vi "Group Tags.vi"(8 "error in (no error)":errorcluster, 10 "Tag Names":string[](array[string]), 11 "Group":string) -> (0 "error out":errorcluster)   [LabVIEW 2010, in "Current Value Table.lvlib"]
doc: "This VI forms a named group which can be used to later read or write data to that entire group. This has the same functionality as including a set of groups during initialization. Tags can be members of multiple groups without issue."
uses:
  Current Value Table.lvlib
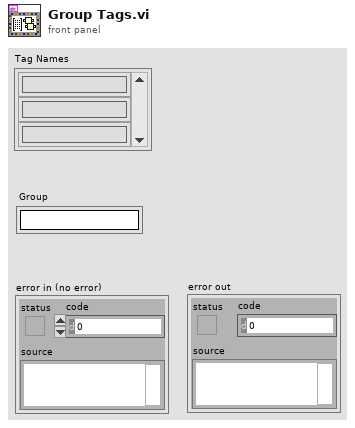
[diagram p1: front panel]
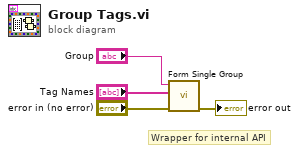
[diagram p0: block diagram]
diagram:
  # "Wrapper for internal API"
  n1 = call "Form Single Group.vi"("error in (no error)"="error in (no error)", "Names"="Tag Names", "Group"="Group") -> ("error out"=→"error out":errorcluster)  [unwired: 8 in]
